vi "read station rs232 port config.vi"(8 "error in":errorcluster, 10 "station idx":i32, 11 "configuration file path in":path) -> (0 "error out":errorcluster, 2 "rs232 port map":T1, 3 "configuration file path out":path)   [LabVIEW 2018]
uses:
  02.Type Def's/station rs232 port map.ctl
  05.UserVI's/file io/ini/type defs/ini file actions.ctl
  05.UserVI's/file io/ini/type defs/ini entry value.ctl
  05.UserVI's/file io/ini/type defs/ini entry types.ctl
  05.UserVI's/file io/ini/type defs/ini entry.ctl
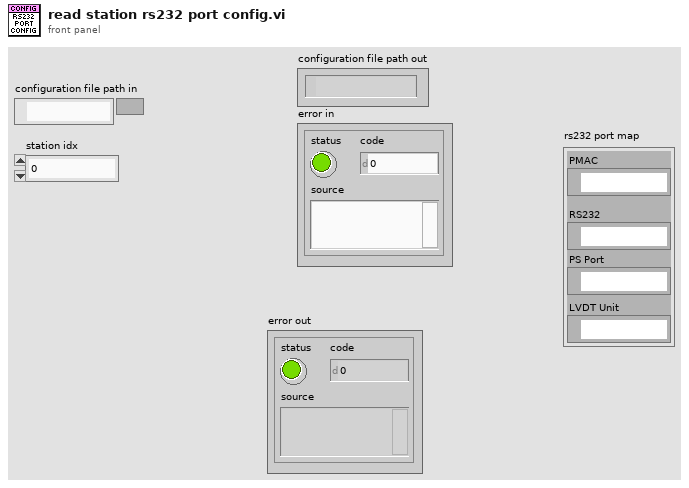
[diagram p1: front panel]
types:
  T1 = typedef "station rs232 port map.ctl" = cluster{"PMAC":refnum<visa-resource-name>, "PS Port":refnum<visa-resource-name>, "LVDT Unit":refnum<visa-resource-name>, "RS232":refnum<visa-resource-name>}
  T2 = typedef "ini entry value.ctl" = cluster{"Boolean":bool, "Dbl":dbl, "I32":i32, "Path":path, "String":string, "U32":u32}
  T3 = typedef "ini file actions.ctl" = enum16{"read ini", "write ini"}
  T4 = typedef "ini entry.ctl" = cluster{"section":string, "key":string, "type":T5, "default value":T2}
  T5 = typedef "ini entry types.ctl" = enum16{"Boolean", "Double", "I32", "Path", "String", "U32"}
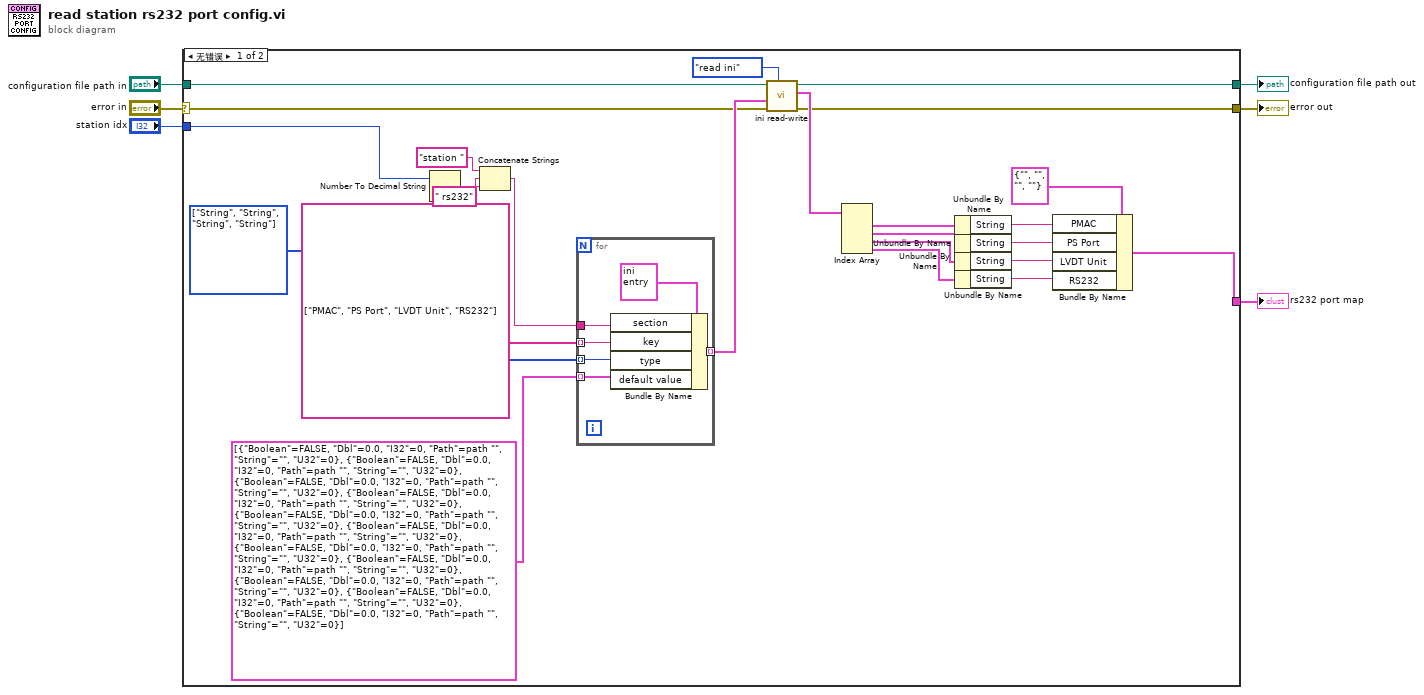
[diagram p0: block diagram]
diagram:
  n1 = case shown="无错误" "error in" {
    selector: "error in" -> [w14 w39]
    tunnel: "configuration file path in" -> [w31 w38]
    tunnel: [w26 w38] -> w5
    tunnel: [w25 w39] -> w4
    tunnel: "station idx" -> [w23 _]
    tunnel: [w11 _] -> w1
    frame No Error {
      w17 = T5[] [enum."String", enum."String", enum."String", enum."String"] items=["Boolean", "Double", "I32", "Path", "String", "U32"]
      n2 = Number To Decimal String(number=w23) -> (decimal integer string=w22:string)  [unwired: 1 in]
      n3 = Concatenate Strings("station ", w22, " rs232" ("string")) -> (w21:string)
      n4 = for {
        tunnel: w21 -> [w36]
        tunnel: string[] ["PMAC", "PS Port", "LVDT Unit", "RS232"] -> [w35] mode=indexing
        tunnel: w17 -> [w34] mode=indexing
        tunnel: T2[] [{"Boolean"=FALSE, "Dbl"=0.0, "I32"=0, "Path"=path "", "String"="", "U32"=0}, {"Boolean"=FALSE, "Dbl"=0.0, "I32"=0, "Path"=path "", "String"="", "U32"=0}, {"Boolean"=FALSE, "Dbl"=0.0, "I32"=0, "Path"=path "", "String"="", "U32"=0}, {"Boolean"=FALSE, "Dbl"=0.0, "I32"=0, "Path"=path "", "String"="", "U32"=0}, {"Boolean"=FALSE, "Dbl"=0.0, "I32"=0, "Path"=path "", "String"="", "U32"=0}, {"Boolean"=FALSE, "Dbl"=0.0, "I32"=0, "Path"=path "", "String"="", "U32"=0}, {"Boolean"=FALSE, "Dbl"=0.0, "I32"=0, "Path"=path "", "String"="", "U32"=0}, {"Boolean"=FALSE, "Dbl"=0.0, "I32"=0, "Path"=path "", "String"="", "U32"=0}, {"Boolean"=FALSE, "Dbl"=0.0, "I32"=0, "Path"=path "", "String"="", "U32"=0}, {"Boolean"=FALSE, "Dbl"=0.0, "I32"=0, "Path"=path "", "String"="", "U32"=0}, {"Boolean"=FALSE, "Dbl"=0.0, "I32"=0, "Path"=path "", "String"="", "U32"=0}] -> [w33] mode=indexing
        tunnel: [w32] -> w15 mode=indexing
        n5 = Bundle By Name(cluster=T4 {"section"="", "key"="", "type"=enum."Boolean", "default value"={"Boolean"=FALSE, "Dbl"=0.0, "I32"=0, "Path"=path "", "String"="", "U32"=0}}, "section"=w36, "key"=w35, "type"=w34, "default value"=w33) -> (w32:T4)
      }
      n6 = call "ini read-write.vi"("action"=ini_file_actions."read ini", "error in (no error)"=w14, "ini entry descriptors"=w15, "configuration file path"=w31) -> ("error out"=w25:errorcluster, "values out"=w29:T2[], "configuration file path out"=w26:path)  [unwired: 5 in]
      n7 = Index Array(array=w29) -> (element #1=w28:T2, element #2=w27:T2, element #3=w20:T2, element #4=w19:T2)  [unwired: 4 in]
      n8 = Unbundle By Name(w28) -> ("String"=w10:string)
      n9 = Unbundle By Name(w27) -> ("String"=w9:string)
      n10 = Unbundle By Name(w20) -> ("String"=w8:string)
      n11 = Unbundle By Name(w19) -> ("String"=w7:string)
      n12 = Bundle By Name(cluster=T1 {"PMAC"="", "PS Port"="", "LVDT Unit"="", "RS232"=""} ("rs232 port map"), "PMAC"=w10, "PS Port"=w9, "LVDT Unit"=w8, "RS232"=w7) -> (w11:T1)
    }
    frame Error {
    }
  }
  "configuration file path out" <- w5
  "error out" <- w4
  "rs232 port map" <- w1
